vi "DSF.Engine.Plugin.Launch Thread.vi"(8 "error in (no error)":errorcluster, 10 "Thread Parameters":refnum<class "Thread Parameters.lvclass">, 11 "Plugin in":refnum<class "Plugin.lvclass">) -> (0 "error out":errorcluster, 2 "Interface":refnum<class "DSF.Engine.Interface.Plugin.lvclass">, 3 "Plugin out":refnum<class "Plugin.lvclass">)   [LabVIEW 2016, in "DSF.Engine.lvlib" / "Plugin.lvclass"]
uses:
  Plugin.lvclass
  Thread Parameters/Thread Parameters.lvclass
  Interface/DSF.Engine.Interface.Plugin.lvclass
  Plugin.lvclass/Plugin.ctl
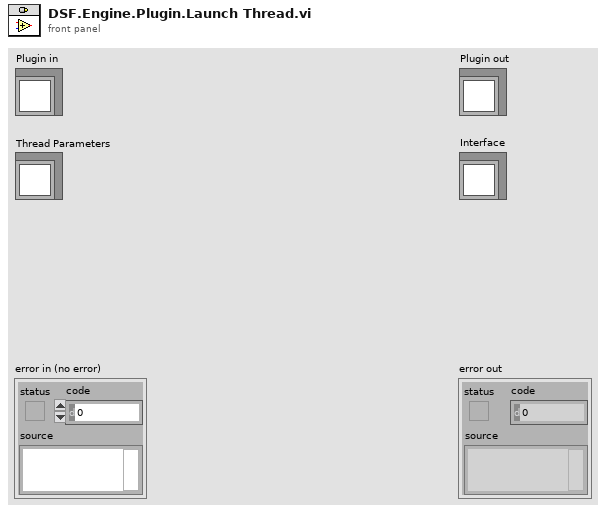
[diagram p1: front panel]
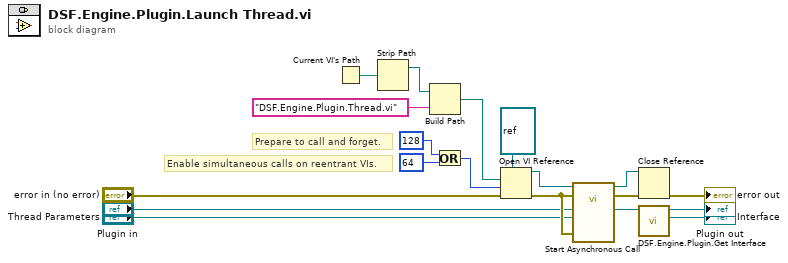
[diagram p0: block diagram]
diagram:
  # "Prepare to call and forget."
  # "Enable simultaneous calls on reentrant VIs."
  n1 = Current VI's Path() -> (path=w18:path)
  n2 = Strip Path(path=w18) -> (stripped path=w17:path)  [unwired: 1 out]
  n3 = Build Path(base path=w17, name or relative path="DSF.Engine.Plugin.Thread.vi") -> (appended path=w10:path)
  n4 = Or(x=128 ("options"), y=64 ("options")) -> (x .or. y?=w4:i32)
  n5 = Open VI Reference(type specifier VI Refnum (for type only)=refnum<vi> refnum, vi path=w10, options=w4, error in (no error)="error in (no error)") -> (vi reference=w13:refnum<vi>, error out=w14:errorcluster)  [unwired: 2 in]
  n6 = call-by-ref "Start Asynchronous Call"(reference=w13, error in=w14, 8:"error in (no error)"=w14, "Thread Parameters"="Thread Parameters", "Plugin in"="Plugin in") -> (reference out=w11:refnum<vi>, error out=w12:errorcluster)  [unwired: 7 in, 2 out]
  n7 = Close Reference(reference=w11, error in (no error)=w12) -> (error out=→"error out":errorcluster)
  n8 = call "DSF.Engine.Plugin.Get Interface.vi"("Plugin in"="Plugin in") -> ("Interface"=→"Interface":refnum<class "DSF.Engine.Interface.Plugin.lvclass">, "Plugin out"=→"Plugin out":refnum<class "Plugin.lvclass">)  [unwired: 9 in]
